vi "parseDataString.vi"(8 "error in (no error)":errorcluster, 9 "OverrideSwapBytes":bool, 10 "Length":i32, 11 "U8ArrayParserAutoIndexing in":refnum<class "U8ArrayParserAutoIndexing.lvclass">) -> (0 "error out":errorcluster, 2 "Data":string, 3 "U8ArrayParserAutoIndexing out":refnum<class "U8ArrayParserAutoIndexing.lvclass">)   [LabVIEW 2016, in "RTUtilities.lvlib" / "U8ArrayParserAutoIndexing.lvclass"]
uses:
  U8ArrayParserAutoIndexing.lvclass
  U8ArrayParserAutoIndexing.lvclass/U8ArrayParserAutoIndexing.ctl
  U8ArrayParser/U8ArrayParserManualIndexing.lvclass
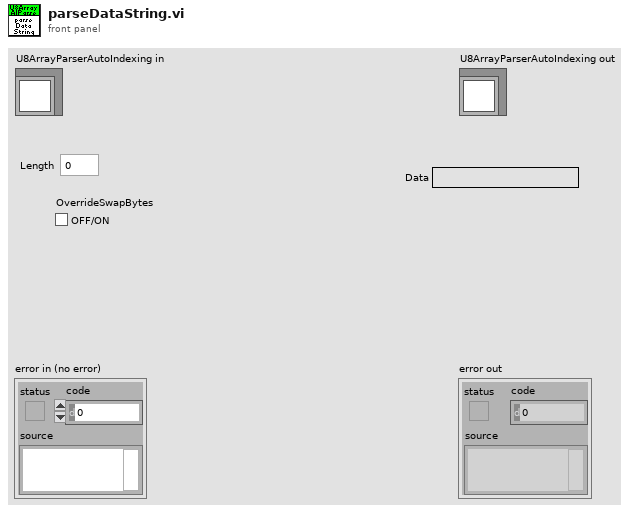
[diagram p1: front panel]
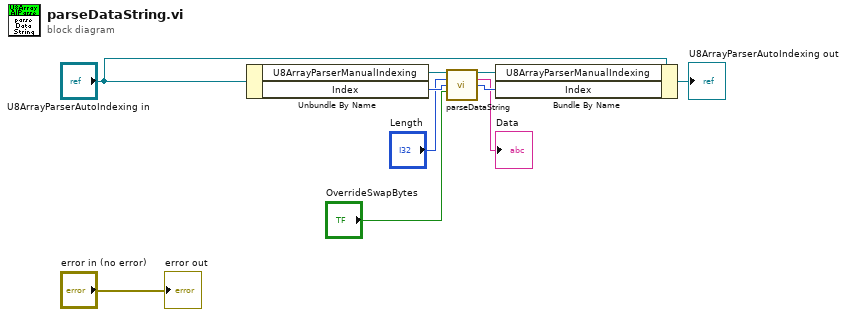
[diagram p0: block diagram]
diagram:
  n1 = Unbundle By Name("U8ArrayParserAutoIndexing in") -> ("U8ArrayParserManualIndexing"=w9:refnum<class "U8ArrayParserManualIndexing.lvclass">, "Index"=w8:i32)
  n2 = call "parseDataString.vi"("U8ArrayParserManualIndexing in"=w9, "Length"="Length", "Index"=w8, "OverrideSwapBytes"="OverrideSwapBytes") -> ("U8ArrayParserManualIndexing out"=w5:refnum<class "U8ArrayParserManualIndexing.lvclass">, "Data"=→"Data":string, "Index out"=w4:i32)  [unwired: 8 in, 1 out]
  n3 = Bundle By Name(cluster="U8ArrayParserAutoIndexing in", "U8ArrayParserManualIndexing"=w5, "Index"=w4) -> (→"U8ArrayParserAutoIndexing out":refnum<class "U8ArrayParserAutoIndexing.lvclass">)
  "error out" <- "error in (no error)"
